vi "2dInterpol.vi"(6 "empty image":bool, 7 "Momentum [MeV/C]":dbl[](array[numeric])=[6.60894171233834, 6.674134434514833, 6.739327156691324, 6.804519878867817, 6.869712601044309, 6.934905323220802, 7.001115808655491, 7.074874289735984, 7.148632770816498, 7.2223912518969975, 7.296149732977504, 7.369908214058004, 7.443666695138518, 7.519431571523783, 7.5994004506796005, 7.679369329835404, 7.759338208991221, 7.839307088147032, 7.919275967302849, 7.999735544885622, 8.08831010924687, 8.176884673608109, 8.265459237969358, 8.354033802330605, 8.442608366691838, 8.536673556671289, 8.638932929286456, 8.741192301901629, 8.843451674516796, 8.945711047131978, 9.046310377133068, 9.14527177158707, 9.24423316604105, 9.343194560495053, 9.442155954949042, 9.548085684765518, 9.662771413739248, 9.777457142712993, 9.892142871686731, 10.007014984780906, 10.12410798402931, 10.24120098327773, 10.358293982526135, 10.475386981774548, 10.61393785885297, 10.757785919121034, 10.901633979389082, 11.045482039657132, 11.189330099925183, 11.333178160193246, 11.477026220461282, 11.621387074621284, 11.765843635222161, 11.910300195823055, 12.054756756423933, 12.199213317024839, 12.343669877625718, 12.48812643822661, 12.65733706497938, 12.828878756230383, 13.000420447481341, 13.171962138732344, 13.343503829983302, 13.516539352320173, 13.706767295375936, 13.896995238431685, 14.08722318148745, 14.277451124543186, 14.467679067598965, 14.674061938688354, 14.884000983932847, 15.093940029177324, 15.303879074421815, 15.514335087940317, 15.733931605172623, 15.953528122404892, 16.17312463963719, 16.392721156869467, 16.641441974942744, 16.91959137343059, 17.197740771918475, 17.475890170406316, 17.736995567132638, 17.996219517127194, 18.255443467121776, 18.514363825911357, 18.76624818908698, 19.018132552262575, 19.270016915438205, 19.521713446226986, 19.77090890391979, 20.02010436161255, 20.269299819305353, 20.51937325739571, 20.784351744604752, 21.04933023181375, 21.31430871902279, 21.57646359532949, 21.83138003043594, 22.086296465542357, 22.34121290064882, 22.593278088764485, 22.840201352843, 23.08712461692149, 23.334047881000004, 23.577351558613884, 23.812441038464108, 24.047530518314325, 24.282619998164517, 24.517620147267404, 24.750965015920844, 24.98430988457432, 25.21765475322776, 25.450999621881234, 25.689195932036494, 25.92888416524386, 26.168572398451193, 26.408260631658553, 26.63426199505935, 26.850827163831255, 27.06739233260312, 27.283957501375017, 27.500522670146886, 27.712720044756068, 27.924798706056684, 28.13687736735733, 28.34895602865794, 28.56269444426666, 28.781218111974976, 28.99974177968332, 29.218265447391637, 29.43678911509998, 29.643616904436016, 29.844957135691793, 30.04629736694754, 30.24763759820332, 30.448977829459068, 30.648608386383984, 30.84755146670724, 31.04649454703052, 31.245437627353777, 31.444380707677055, 31.64107443732088, 31.836738432664735, 32.03240242800857, 32.228066423352416, 32.423730418696245, 32.62397485791499, 32.827611601904195, 33.03124834589337, 33.23488508988257, 33.43852183387175, 33.63428761070054, 33.826056513686936, 34.01782541667336, 34.209594319659764, 34.40136322264619, 34.59110928959807, 34.778363125774824, 34.96561696195154, 35.15287079812829, 35.34012463430501, 35.52714731647596, 35.712243022468655, 35.897338728461364, 36.08243443445405, 36.26753014044676, 36.45262584643944, 36.63597843369212, 36.818597951056496, 37.00121746842091, 37.18383698578529, 37.366456503149706, 37.54854552304384, 37.72883386123314, 37.90912219942242, 38.08941053761173, 38.269698875801005, 38.449987213990305, 38.629470572090156, 38.808575796219266, 38.987681020348354, 39.166786244477464, 39.345891468606546, 39.52484664648395, 39.702398608284796, 39.879950570085654, 40.05750253188649, 40.23505449368736, 40.41260645548822, 40.58945026751812, 40.7654760131042, 40.94150175869025, 41.117527504276325, 41.29355324986238, 41.46957899544846, 41.644751338769616, 41.81968655831688, 41.99462177786413, 42.169556997411405, 42.344492216958656, 42.51875693951674, 42.68349222118452, 42.84822750285234, 43.01296278452012, 43.17769806618792, 43.34243334785571, 43.50716862952352, 43.679886334776235, 43.85264443141208, 44.025402528047906, 44.198160624683744, 44.37091872131957, 44.54348995847316, 44.71534154718959, 44.88719313590604, 45.05904472462247, 45.23089631333892, 45.402747902055346, 45.57062771212531, 45.732210582629754, 45.89379345313423, 46.05537632363868, 46.21695919414316, 46.37854206464761, 46.541815635463166, 46.71195356700807, 46.882091498552995, 47.05222943009789, 47.22236736164282, 47.39250529318772, 47.55935369809548, 47.71920204761723, 47.87905039713896, 48.03889874666071, 48.198747096182444, 48.35859544570419, 48.51900732670278, 48.68774294895169, 48.85647857120057, 49.02521419344947, 49.19394981569835, 49.362685437947256, 49.53001633617772, 49.68847283259404, 49.84692932901034, 50.00538582542666, 50.16384232184296, 50.322298818259284, 50.480755314675584, 50.64138689181567, 50.80247841452205, 50.96356993722844, 51.12466145993481, 51.285752982641206, 51.446844505347585, 51.60793602805398, 51.76902755076034, 51.93011907346675, 52.09121059617312, 52.25230211887951, 52.41339364158589, 52.574485164292284, 52.73557668699865, 52.89666820970505, 53.05615668072052, 53.2120019934137, 53.36784730610686, 53.52369261880004, 53.67953793149321, 53.83538324418639, 53.99122855687955, 54.147073869572736, 54.30291918226592, 54.458764494959084, 54.614609807652265, 54.770455120345424, 54.926300433038605, 55.08214574573177, 55.23799105842495, 55.39383637111811, 55.549331749692385, 55.70384805026412, 55.858364350835885, 56.01288065140763, 56.16739695197938, 56.32191325255112, 56.476429553122884, 56.63094585369462, 56.78546215426638, 56.93997845483812, 57.094494755409876, 57.24901105598161, 57.40352735655338, 57.55804365712512, 57.712559957696875, 57.86707625826862, 58.02118353433666, 58.17077938929847, 58.3203752442603, 58.4699710992221, 58.61956695418394, 58.76916280914574, 58.918758664107564, 59.06835451906938, 59.2179503740312, 59.367546228993014, 59.51714208395484, 59.66673793891665, 59.81633379387848, 59.96592964884028, 60.11552550380211, 60.26512135876392, 60.41471721372575, 60.56391073898331, 60.7124216000462, 60.860932461109115, 61.00944332217201, 61.15795418323492, 61.30646504429782, 61.45497590536073, 61.60348676642363, 61.751997627486546, 61.900508488549434, 62.049019349612344, 62.19753021067524, 62.346041071738156, 62.49455193280105, 62.64306279386397, 62.79157365492685, 62.94008451598977, 63.086056420086244, 63.229834378343355, 63.37361233660046, 63.517390294857584, 63.66116825311469, 63.8049462113718, 63.9487241696289, 64.09250212788602, 64.23628008614313, 64.38005804440024, 64.52383600265736, 64.66761396091447, 64.81139191917158, 64.95516987742869, 65.0989478356858, 65.24272579394291, 65.38650375220003, 65.52960640229915, 65.66882073254745, 65.80803506279574, 65.94724939304405, 66.08646372329234, 66.22567805354063, 66.36489238378893, 66.50410671403723, 66.64332104428553, 66.78253537453382, 66.92174970478213, 67.06096403503042, 67.20017836527872, 67.33939269552701, 67.4786070257753, 67.6178213560236, 67.75703568627189, 67.89625001652018, 68.03528972211087, 68.17358269798136, 68.31187567385186, 68.45016864972236, 68.58846162559284, 68.72675460146334, 68.86504757733384, 69.00334055320432, 69.14163352907482, 69.27992650494531, 69.41821948081582, 69.5565124566863, 69.6948054325568, 69.83309840842729, 69.97139138429779, 70.10968436016829, 70.24797733603877, 70.38627031190927, 70.52408326957418, 70.65807020581502, 70.79205714205587, 70.92604407829671, 71.06003101453756, 71.19401795077839, 71.32800488701923, 71.46199182326008, 71.59597875950092, 71.72996569574175, 71.8639526319826, 71.99793956822344, 72.13192650446427, 72.26591344070512, 72.39990037694596, 72.53388731318681, 72.66787424942765, 72.80186118566849, 72.93584812190933, 73.06796710164868, 73.1978256146809, 73.32768412771311, 73.45754264074534, 73.58740115377758, 73.7172596668098, 73.84711817984201, 73.97697669287425, 74.10683520590648, 74.2366937189387, 74.36655223197091, 74.49641074500315, 74.62626925803536, 74.7561277710676, 74.88598628409983, 75.01584479713206, 75.14570331016428, 75.2755618231965, 75.40542033622873, 75.53448281537831, 75.66036684360022, 75.78625087182209, 75.91213490004398, 76.03801892826587, 76.16390295648776, 76.28978698470965, 76.41567101293154, 76.54155504115342, 76.6674390693753, 76.7933230975972, 76.91920712581909, 77.04509115404097, 77.17097518226286, 77.29685921048474, 77.42274323870663, 77.54862726692852, 77.67451129515042, 77.8003953233723, 77.92627935159419, 78.05089864346074, 78.17306614207223, 78.2952336406837, 78.4174011392952, 78.53956863790668, 78.66173613651816, 78.78390363512965, 78.90607113374112, 79.02823863235261, 79.1504061309641, 79.27257362957558, 79.39474112818706, 79.51690862679855, 79.63907612541003, 79.76124362402152, 79.88341112263299, 80.00557862124448, 80.12774611985597, 80.24991361846746, 80.37208111707893, 80.49424861569042, 80.61583187133728, 80.73733255294418, 80.8588332345511, 80.98033391615802, 81.10183459776492, 81.22333527937184, 81.34483596097876, 81.46633664258566, 81.58783732419256, 81.70933800579948, 81.8308386874064, 81.9523393690133, 82.07384005062022, 82.19534073222714, 82.31684141383404, 82.43834209544096, 82.55984277704788, 82.68134345865478, 82.8028441402617, 82.92434482186862, 83.04394729047074, 83.15911526152681, 83.27428323258286, 83.38945120363893, 83.504619174695, 83.61978714575105, 83.73495511680711, 83.85012308786318, 83.96529105891923, 84.0804590299753, 84.19562700103137, 84.31079497208742, 84.42596294314349, 84.54113091419956, 84.65629888525561, 84.77146685631168, 84.88663482736773, 85.0018027984238, 85.11697076947986, 85.23213874053593, 85.347306711592, 85.46247468264805, 85.57422059963754, 85.68360732902616, 85.79299405841478, 85.9023807878034, 86.01176751719201, 86.12115424658063, 86.23054097596925], 9 "pixel angle (y)":dbl[](array[numeric]), 10 "Y angles 2D":dbl[][](graph), 11 "Z":dbl[][](graph)) -> (0 "Sum Y":cluster{"Ramp Pattern":dbl[], dbl[]}, 1 "spec cluster 2":cluster{"Momentum [MeV/C]":dbl[], dbl[]}(graph), 5 "time: 2Dinter":u32)   [LabVIEW 2011]
uses:
  NI_AALBase.lvlib
  NI_AALPro.lvlib
  NI_Gmath.lvlib
panel:
  in  "error out":errorcluster
  out "error":i32
  out "size(s) 3":i32[](array[numeric])
  out "size(s) 2":i32[](array[numeric])
  out "size(s)":i32[](array[numeric])
  out "time: spectra":u32
  out "time: prepare arrays":u32
  out "charge (YSum)":dbl format="%0.4f"
  out "charge (spectra)":dbl format="%0.4f"
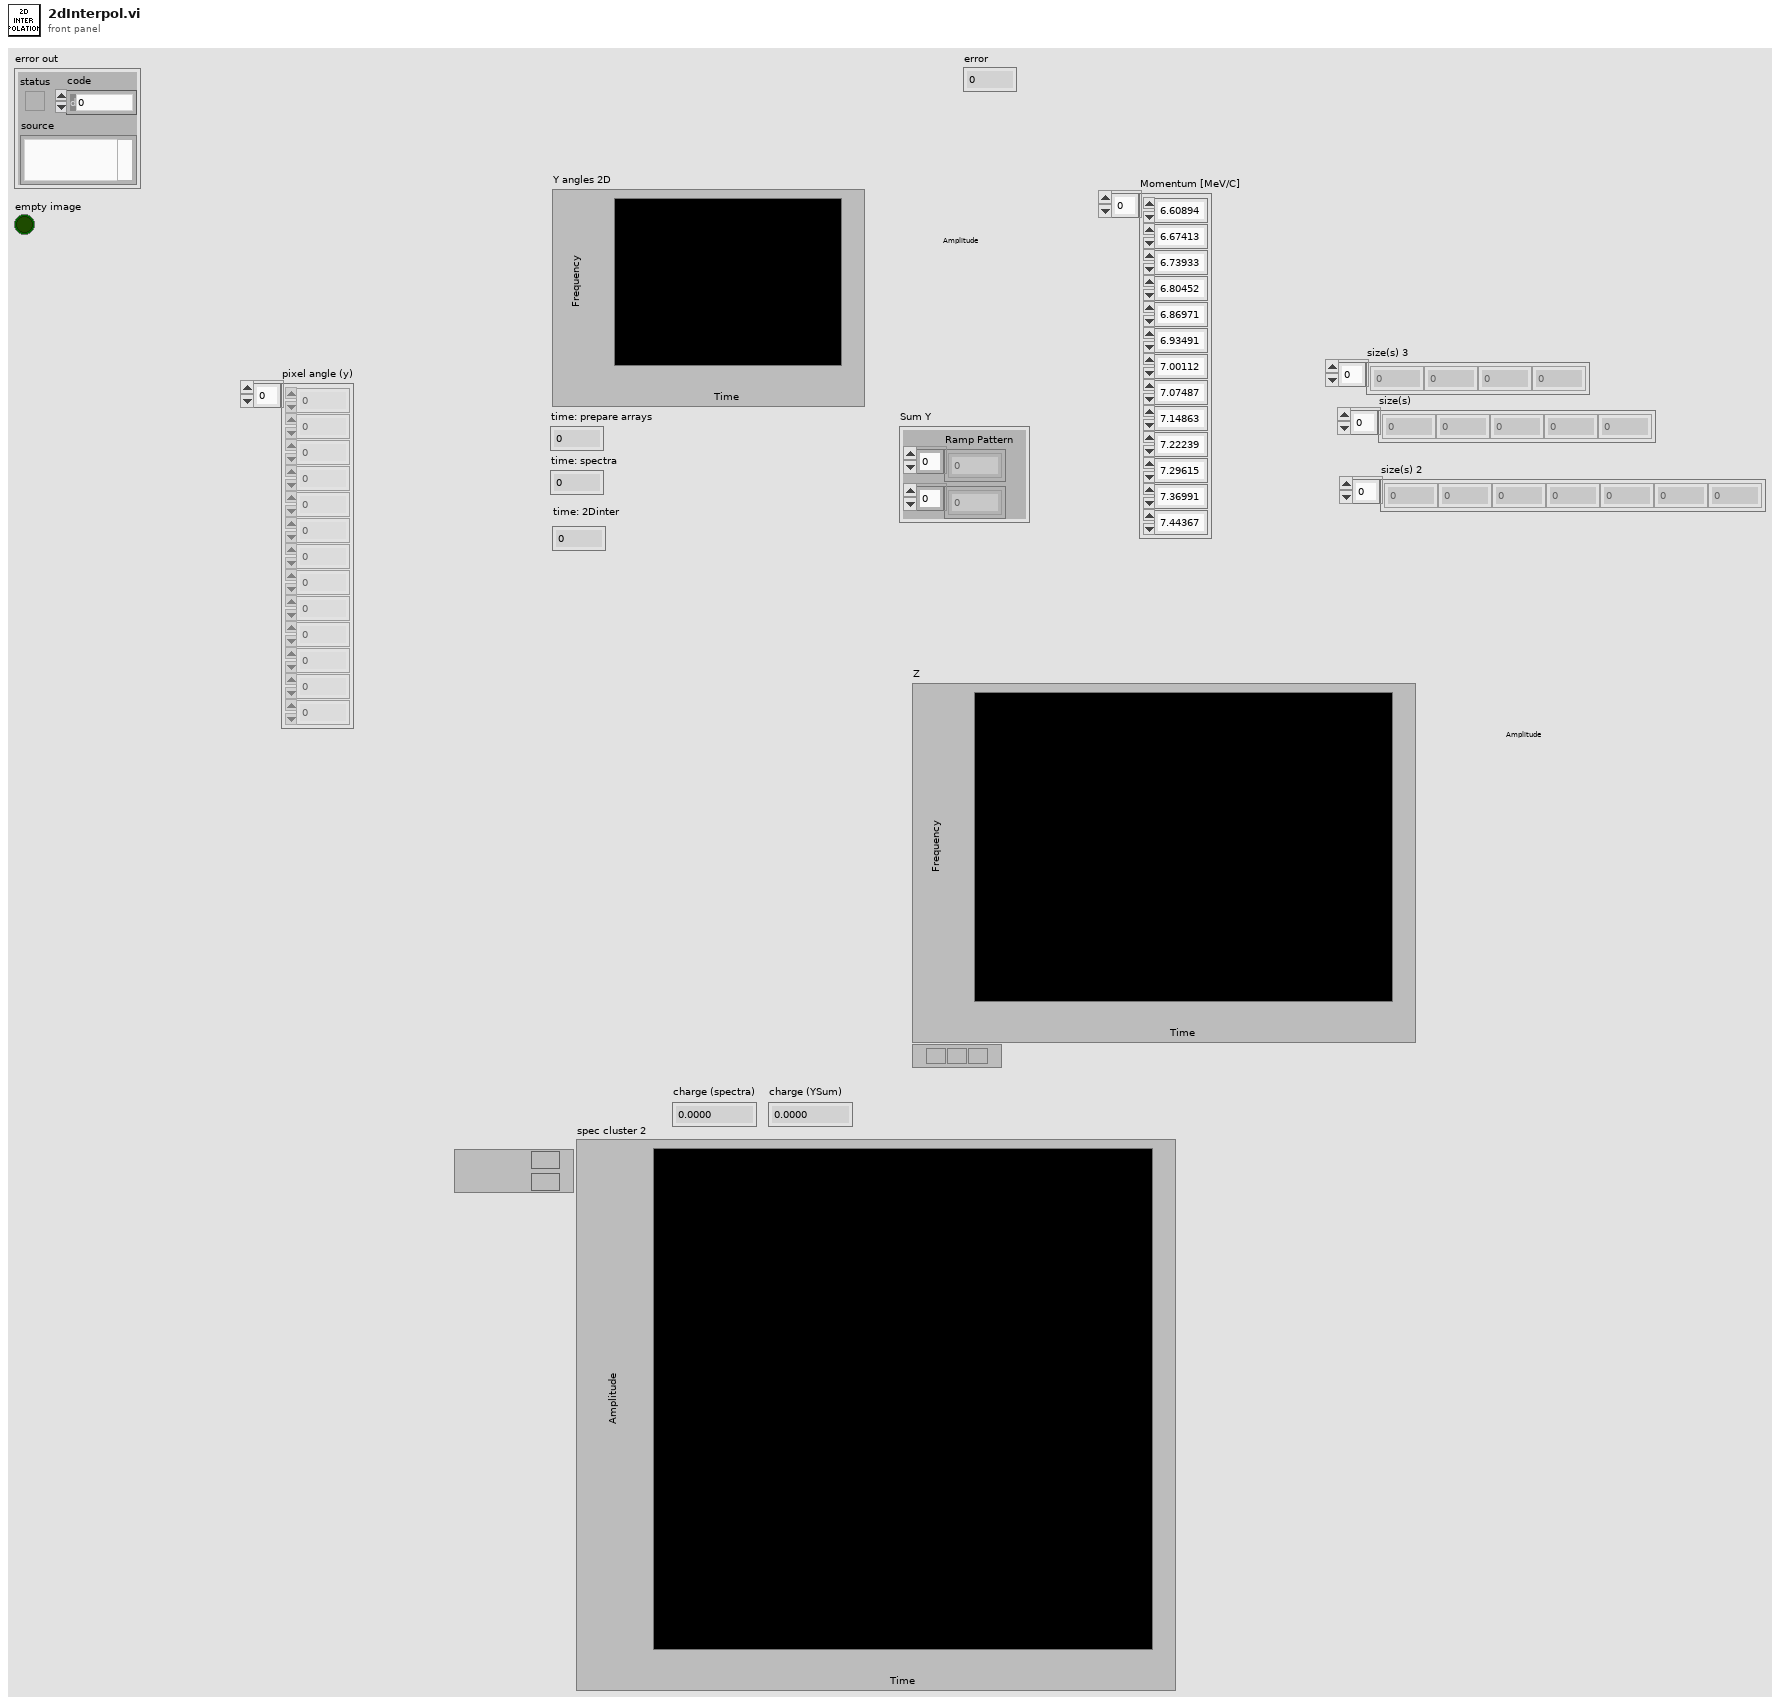
[diagram p1: front panel]
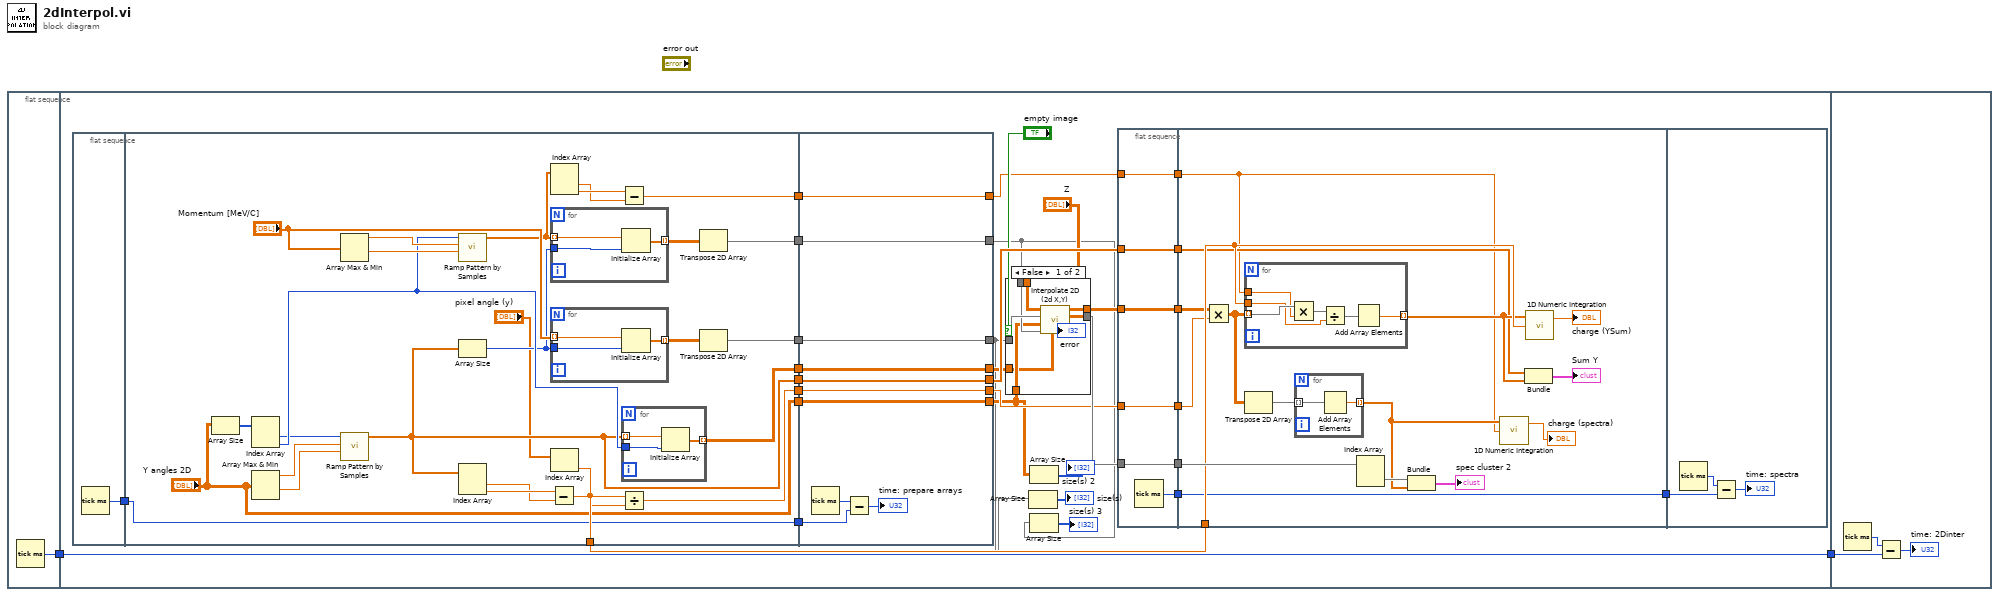
[diagram p0: block diagram]
diagram:
  n1 = flat-sequence {
    tunnel: [w3] -> w2
    tunnel: w2 -> [w35]
    tunnel: [w35] -> w1
    tunnel: w1 -> [w127]
    frame #0 {
      n2 = Tick Count (ms)() -> (millisecond timer value=w3:u32)
    }
    frame #1 {
      n3 = flat-sequence {
        tunnel: [w79] -> w21
        tunnel: [w87] -> w33
        tunnel: [w104] -> w28
        tunnel: [w97] -> w27
        tunnel: [w88] -> w26
        tunnel: [w86] -> w25
        tunnel: [w85] -> w24
        tunnel: ["Y angles 2D"] -> w23
        tunnel: [w81] -> w22
        tunnel: w21 -> [w80]
        tunnel: [w80] -> w20
        tunnel: [w119] -> w29
        tunnel: [w120] -> w9
        tunnel: [w121] -> w30
        tunnel: [w122] -> w32
        tunnel: [w123] -> w12
        tunnel: [w124] -> w7
        tunnel: [w125] -> w8
        tunnel: w28 -> [w125]
        tunnel: w27 -> [w124]
        tunnel: w26 -> [w123]
        tunnel: w25 -> [w122]
        tunnel: w24 -> [w121]
        tunnel: w23 -> [w120]
        tunnel: w22 -> [w119]
        tunnel: w20 -> [w117]
        frame #0 {
          n4 = Tick Count (ms)() -> (millisecond timer value=w79:u32)
        }
        frame #1 {
          n5 = Array Size(array="Y angles 2D") -> (size(s)=w106:i32[])
          n6 = Index Array(array=w106) -> (element #1=w92:i32, element #2=w96:i32)  [unwired: 2 in]
          n7 = Array Max & Min(array="Y angles 2D") -> (max value=w100:dbl, min value=w99:dbl)  [unwired: 2 out]
          n8 = Array Max & Min(array="Momentum [MeV/C]") -> (max value=w103:dbl, min value=w102:dbl)  [unwired: 2 out]
          n9 = call "Ramp Pattern by Samples.vi"("start"=w99, "end"=w100, "samples"=w92) -> ("Ramp Pattern"=w86:dbl[])  [unwired: 7 in, 1 out]
          n10 = call "Ramp Pattern by Samples.vi"("start"=w102, "end"=w103, "samples"=w96) -> ("Ramp Pattern"=w91:dbl[])  [unwired: 7 in, 1 out]
          n11 = Array Size(array=w86) -> (size(s)=w93:i32)
          n12 = Index Array(array=w86) -> (element #1=w94:dbl, element #2=w95:dbl)  [unwired: 2 in]
          n13 = Subtract(x=w95, y=w94) -> (x-y=w87:dbl)
          n14 = Index Array(array=w91) -> (element #1=w89:dbl, element #2=w90:dbl)  [unwired: 2 in]
          n15 = for {
            tunnel: w91 -> [w112] mode=indexing
            tunnel: w93 -> [w111]
            tunnel: [w110] -> w101 mode=indexing
            n16 = Initialize Array(w112, w111) -> (w110:dbl[])
          }
          n17 = for {
            tunnel: "Momentum [MeV/C]" -> [w115] mode=indexing
            tunnel: w93 -> [w114]
            tunnel: [w113] -> w105 mode=indexing
            n18 = Initialize Array(w115, w114) -> (w113:dbl[])
          }
          n19 = Index Array(array="pixel angle (y)") -> (element=w84:dbl)  [unwired: 1 in]
          n20 = Subtract(x=w90, y=w89) -> (x-y=w88:dbl)
          n21 = Divide(x=w87, y=w84) -> (x/y=w85:dbl)
          n22 = for {
            tunnel: w86 -> [w109] mode=indexing
            tunnel: w96 -> [w108]
            tunnel: [w107] -> w81 mode=indexing
            n23 = Initialize Array(w109, w108) -> (w107:dbl[])
          }
          n24 = Transpose 2D Array(2D array=w101) -> (transposed array=w97:dbl[][])
          n25 = Transpose 2D Array(2D array=w105) -> (transposed array=w104:dbl[][])
        }
        frame #2 {
          n26 = Tick Count (ms)() -> (millisecond timer value=w118:u32)
          n27 = Subtract(x=w118, y=w117) -> (x-y=→"time: prepare arrays":u32)
        }
      }
      n28 = case shown="False" "empty image" {
        tunnel: w8 -> [w43 _]
        tunnel: [w42 w44] -> w34
        tunnel: w7 -> [w41 w44]
        tunnel: "Z" -> [w40 w45]
        tunnel: [w39 w45] -> w31
        tunnel: w9 -> [w38 _]
        tunnel: w29 -> [w37 _]
        frame False {
          n29 = call "Interpolate 2D (2d X,Y).vi"("yi"=w37, "xi"=w41, "Y"=w38, "X"=w43, "Z"=w40) -> ("error"=→"error":i32, "xi used"=w42:dbl[][], "zi"=w39:dbl[][])  [unwired: 3 in, 1 out]
        }
        frame True {
        }
      }
      n30 = Array Size(array=w8) -> (size(s)=→"size(s)":i32[])
      n31 = Array Size(array=w9) -> (size(s)=→"size(s) 2":i32[])
      n32 = Array Size(array=w7) -> (size(s)=→"size(s) 3":i32[])
      n33 = flat-sequence {
        tunnel: w30 -> [w48]
        tunnel: w31 -> [w49]
        tunnel: w32 -> [w50]
        tunnel: w34 -> [w51]
        tunnel: [w51] -> w19
        tunnel: [w50] -> w18
        tunnel: [w49] -> w17
        tunnel: [w48] -> w16
        tunnel: [w47] -> w15
        tunnel: w12 -> [w46]
        tunnel: [w46] -> w11
        tunnel: w33 -> [w60]
        tunnel: w19 -> [w65]
        tunnel: w18 -> [w58]
        tunnel: w17 -> [w56]
        tunnel: w16 -> [w55]
        tunnel: w15 -> [w53]
        tunnel: [w53] -> w14
        tunnel: w11 -> [w52]
        tunnel: w14 -> [w77]
        frame #0 {
          n34 = Tick Count (ms)() -> (millisecond timer value=w47:u32)
        }
        frame #1 {
          n35 = Multiply(x=w56, y=w55) -> (x*y=w54:dbl[][])
          n36 = for {
            tunnel: w54 -> [w74] mode=indexing
            tunnel: [w75] -> w59 mode=indexing
            tunnel: w52 -> [w73]
            tunnel: w60 -> [w71]
            n37 = Multiply(x=w74, y=w73) -> (x*y=w72:dbl[])
            n38 = Divide(x=w72, y=w71) -> (x/y=w70:dbl[])
            n39 = Add Array Elements(numeric array=w70) -> (sum=w75:dbl)
          }
          n40 = Transpose 2D Array(2D array=w54) -> (transposed array=w67:dbl[][])
          n41 = for {
            tunnel: w67 -> [w68] mode=indexing
            tunnel: [w69] -> w63 mode=indexing
            n42 = Add Array Elements(numeric array=w68) -> (sum=w69:dbl)
          }
          n43 = Index Array(array=w65) -> (element=w64:dbl[])  [unwired: 2 in]
          n44 = Bundle("xi used"=w64, w63) -> (→"spec cluster 2":cluster{"xi used":dbl[], dbl[]})  [unwired: 1 in]
          n45 = call "1D Numeric Integration.vi"("dt"=w52, "Input Array"=w63) -> ("result"=→"charge (spectra)":dbl)  [unwired: 1 in, 1 out]
          n46 = Bundle("Ramp Pattern"=w58, w59) -> (→"Sum Y":cluster{"Ramp Pattern":dbl[], dbl[]})  [unwired: 1 in]
          n47 = call "1D Numeric Integration.vi"("dt"=w60, "Input Array"=w59) -> ("result"=→"charge (YSum)":dbl)  [unwired: 1 in, 1 out]
        }
        frame #2 {
          n48 = Tick Count (ms)() -> (millisecond timer value=w78:u32)
          n49 = Subtract(x=w78, y=w77) -> (x-y=→"time: spectra":u32)
        }
      }
    }
    frame #2 {
      n50 = Tick Count (ms)() -> (millisecond timer value=w128:u32)
      n51 = Subtract(x=w128, y=w127) -> (x-y=→"time: 2Dinter":u32)
    }
  }
